vi "Write Get Connection List Msg.vi"(10 "Connection Listener.lvlib:Get Connection List Msg.lvclass":refnum<class "Get Connection List Msg.lvclass">=refnum, 11 "Connection Listener in":refnum<class "Connection Listener.lvclass">) -> (3 "Connection Listener out":refnum<class "Connection Listener.lvclass">)   [LabVIEW 2017, in "Connection Listener.lvlib" / "Connection Listener.lvclass"]
uses:
  Connection Listener.lvclass
  Connection Listener Messages/Get Connection List Msg/Get Connection List Msg.lvclass
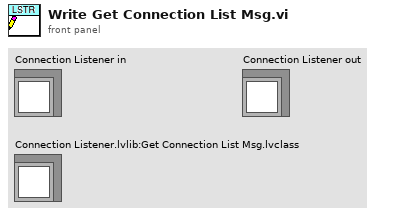
[diagram p1: front panel]
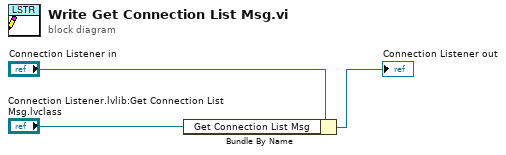
[diagram p0: block diagram]
diagram:
  n1 = Bundle By Name(cluster="Connection Listener in", "Get Connection List Msg"="Connection Listener.lvlib:Get Connection List Msg.lvclass") -> (→"Connection Listener out":refnum<class "Connection Listener.lvclass">)
